vi "ex4-11.vi"   [LabVIEW 2009]
uses:
  <vilib>/NXT/Subs/MotorOutput.ctl
  <vilib>/NXT/Dual Mode Library/Motors/MotorBrake.vi
  <vilib>/NXT/Dual Mode Library/Waits/Wait_Num.vi
  <vilib>/NXT/Dual Mode Library/Motors/MotorOn.vi
  <vilib>/NXT/Dual Mode Library/Motors/ResetMotor.vi
  <vilib>/NXT/Dual Mode Library/Waits/Wait_Rotation.vi
  <vilib>/NXT/Dual Mode Library/Motors/MotorReverse.vi
types:
  T1 = typedef "MotorOutput.ctl" = u8
  T2 = typedef "LVHSConnector.ctl" = cluster{"error":errorcluster, "address":string, "NXT #":i32, "Show Error":bool, "Connection":u16}
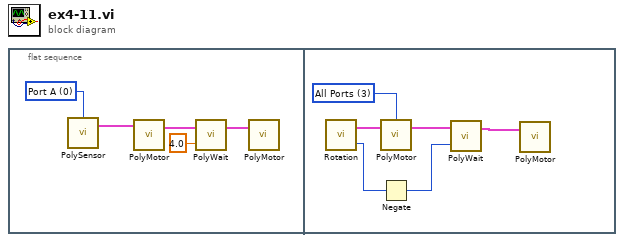
[diagram p0: block diagram]
diagram:
  n1 = flat-sequence {
    frame #0 {
      w2 = T1 0 items=["Port A", "Port B", "Port C", "All Ports"] ("Port (All Ports)")
      n2 = call-poly <vilib>:"PolySensor.vi"("Port (All Ports)"=w2) -> ("NXT"=w3:T2)  [unwired: 3 in]
      n3 = call-poly <vilib>:"PolyMotor.vi"("NXT"=w3) -> ("NXT"=w5:T2)  [unwired: 3 in]
      n4 = call-poly <vilib>:"PolyWait.vi"("Time (1 sec)"=sgl 4.0, "NXT"=w5) -> ("NXT"=w4:T2)  [unwired: 2 in]
      n5 = call-poly <vilib>:"PolyMotor.vi"("NXT"=w4) -> ()  [unwired: 3 in, 1 out]
    }
    frame #1 {
      w8 = T1 3 items=["Port A", "Port B", "Port C", "All Ports"] ("Output Port (All Ports)")
      n6 = call <vilib>:"Rotation.vi"() -> ("Rotation"=w7:i32, "NXT"=w11:T2)  [unwired: 3 in]
      n7 = call-poly <vilib>:"PolyMotor.vi"("NXT"=w11, "Output Port (All Ports)"=w8) -> ("NXT"=w10:T2)  [unwired: 2 in]
      n8 = Negate(x=w7) -> (-x=w6:i32)
      n9 = call-poly <vilib>:"PolyWait.vi"("Position Change (180)"=w6, "NXT"=w10) -> ("NXT"=w9:T2)  [unwired: 2 in]
      n10 = call-poly <vilib>:"PolyMotor.vi"("NXT"=w9) -> ()  [unwired: 3 in, 1 out]
    }
  }
